vi "Encoder.vi"(0 "Serial Port in":refnum<visa-resource-name>, 1 "simulate?":bool, 3 "error in":errorcluster, 4 "pulses":u32) -> (5 "Serial Port out":refnum<visa-resource-name>, 6 "status":T1, 7 "error out":errorcluster)   [LabVIEW 2011]
doc: "Reads the HEDS-9140 angular position encoder connected via Arduino through the given serial connection (USB-tunneled).\nWants the number of pulses per revolution on the encoder artwork.\nReturns a cluster containing the current position (ie pulse count), velocity (puses/s), angle (°), and three bool flags:\n- home? (if true, homing has been done)\n- new? (if true, this is a new data, ie the encoder was moved since tha last reading)\n- reset? (if true, the 0 position has been passed and this is a new revolution)"
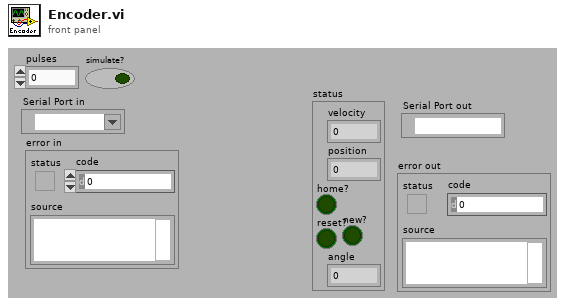
[diagram p1: front panel]
types:
  T1 = cluster{"velocity":dbl, "position":u32, "home?":bool, "reset?":bool, "angle":dbl, "new?":bool}
  T2 = cluster{"[0]":dbl, "[1]":dbl, "[2]":dbl, "[3]":dbl}
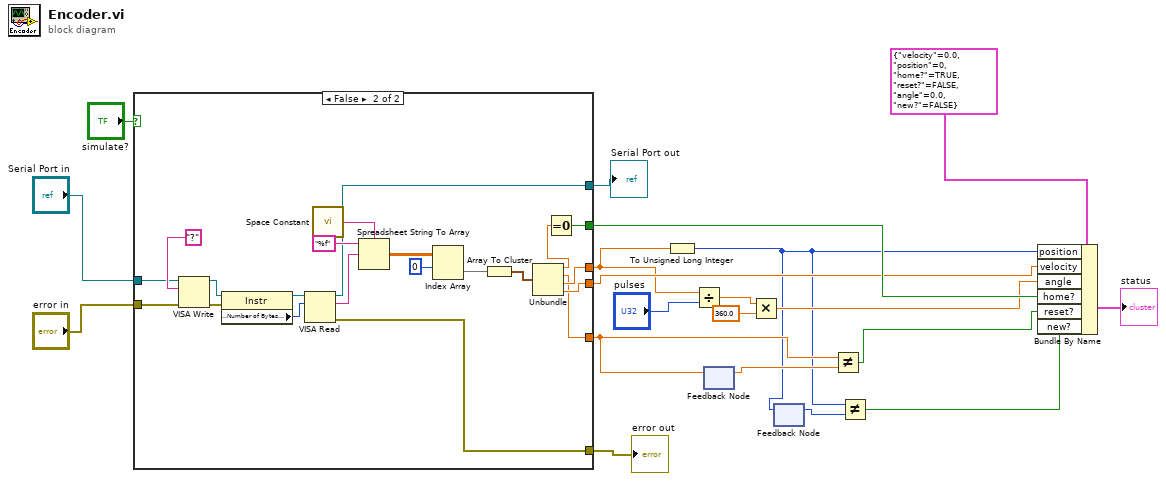
[diagram p0: block diagram]
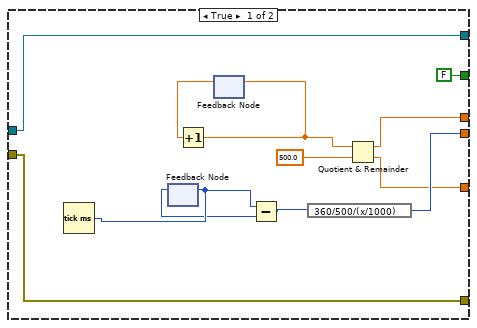
[diagram p2: hidden frame]
diagram:
  n1 = case shown="False" "simulate?" {
    tunnel: [w28 w34] -> w5
    tunnel: [w23 w35] -> w6
    tunnel: [w31 w45] -> w20
    tunnel: "error in" -> [w31 w42]
    tunnel: "Serial Port in" -> [w32 w41]
    tunnel: [w32 w40] -> w17
    tunnel: [FALSE w37] -> w11
    tunnel: [w21 w33] -> w13
    frame True {
      n2 = Tick Count (ms)() -> (millisecond timer value=w27:u32)
      n3 = feedback-in #1(w27) -> ()
      n4 = feedback #1() -> (w26:u32)  [unwired: 1 in]
      n5 = feedback #2() -> (w30:dbl)  [unwired: 1 in]
      n6 = Increment(x=w30) -> (x+1=w29:dbl)
      n7 = feedback-in #2(w29) -> ()
      n8 = Subtract(x=w27, y=w26) -> (x-y=w24:u32)
      n9 = expression code="360/500/(x/1000)"(w24) -> (w23:u32)
      n10 = Quotient & Remainder(x=w29, y=500.0) -> (x-y*floor(x/y)=w28:dbl, floor(x/y)=w21:dbl)
    }
    frame False {
      n11 = VISA Write(VISA resource name=w41, write buffer="?", error in (no error)=w42) -> (VISA resource name out=w43:refnum<visa-resource-name>, error out=w46:errorcluster)  [unwired: 1 out]
      n12 = property class="Instr"(reference=w43, error in=w46) -> (reference out=w44:refnum<visa-resource-name>, "Serial Settings:Number of Bytes at Serial Port"=w39:u32)  [unwired: 1 out]
      n13 = VISA Read(VISA resource name=w44, byte count=w39) -> (VISA resource name out=w40:refnum<visa-resource-name>, read buffer=w50:string, error out=w45:errorcluster)  [unwired: 1 in, 1 out]
      n14 = call <vilib>:"Space Constant.vi"() -> ("String"=w48:string)
      n15 = Spreadsheet String To Array(delimiter (Tab)=w48, format string="%f" ("spreadsheet string"), spreadsheet string=w50) -> (array=w51:dbl[][])  [unwired: 1 in]
      n16 = Index Array(array=w51, index (row)=0) -> (element=w53:dbl[])  [unwired: 1 in]
      n17 = Array To Cluster(array=w53) -> (cluster=w36:T2)
      n18 = Unbundle(w36) -> ("[0]"=w38:dbl, "[1]"=w33:dbl, "[2]"=w34:dbl, "[3]"=w35:dbl)
      n19 = Equal To 0?(x=w38) -> (x = 0?=w37:bool)
    }
  }
  "error out" <- w20
  "Serial Port out" <- w17
  n20 = To Unsigned Long Integer(number=w5) -> (unsigned 32bit integer=w2:u32)
  n21 = Divide(x=w5, y="pulses") -> (x/y=w8:dbl)
  n22 = feedback-in #3(w13) -> ()
  n23 = feedback #3() -> (w14:dbl)  [unwired: 1 in]
  n24 = Multiply(x=w8, y=360.0) -> (x*y=w7:dbl)
  n25 = feedback #4() -> (w3:u32)  [unwired: 1 in]
  n26 = feedback-in #4(w2) -> ()
  n27 = Not Equal?(x=w13, y=w14) -> (x != y?=w12:bool)
  n28 = Not Equal?(x=w2, y=w3) -> (x != y?=w1:bool)
  n29 = Bundle By Name(cluster=T1 {"velocity"=0.0, "position"=0, "home?"=TRUE, "reset?"=FALSE, "angle"=0.0, "new?"=FALSE}, "position"=w2, "velocity"=w6, "angle"=w7, "home?"=w11, "reset?"=w12, "new?"=w1) -> (→"status":T1)
